vi "ParseXMLRPC.vi"(8 "Parsed In":string, 11 "XML In":string) -> (0 "Parsed Out":string, 3 "XML Out":string)   [LabVIEW 2012]
panel:
  # "<value><array><data>\n  <value>test</value>\n  <value><boolean>1</boolean></value>\n</data></array></value>"
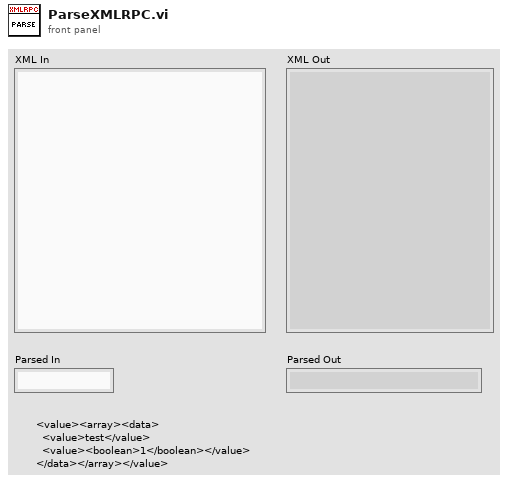
[diagram p1: front panel]
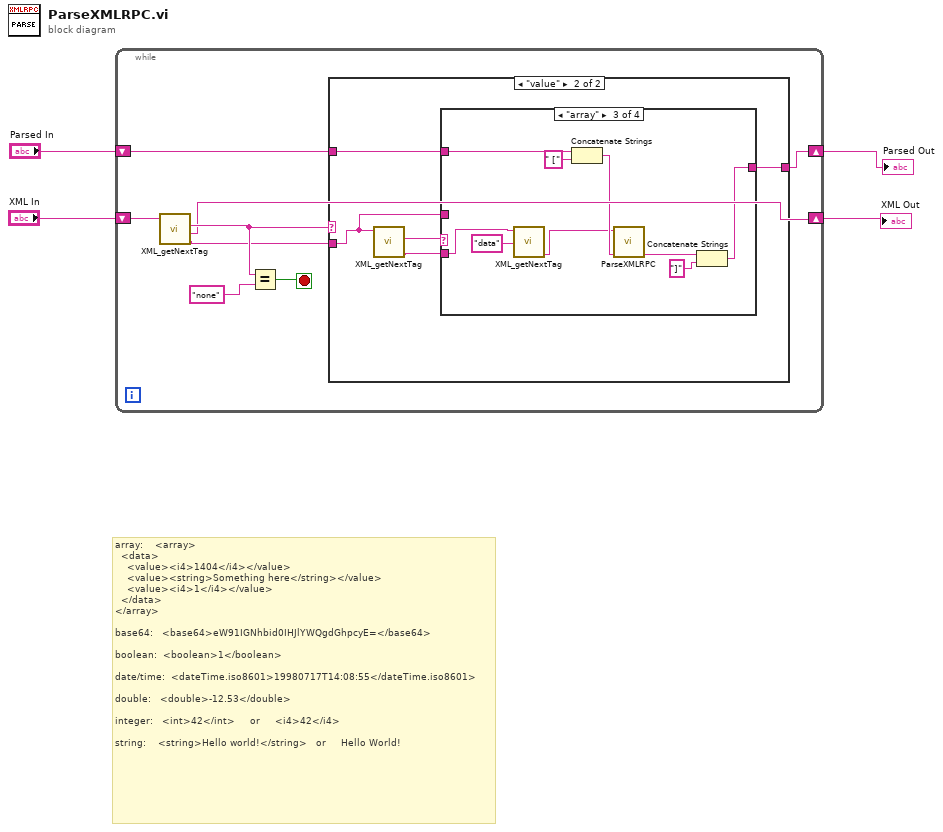
[diagram p0: block diagram]
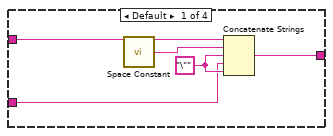
[diagram p3: hidden frame]
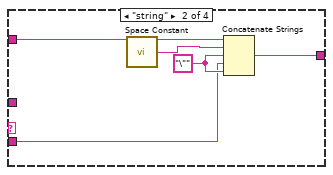
[diagram p4: hidden frame]
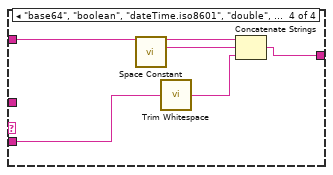
[diagram p5: hidden frame]
diagram:
  # "array:    <array>\n  <data>\n    <value><i4>1404</i4></value>\n    <value><string>Something here</string></value>\n    <value><i4>1</i4></value>\n  </data>\n</array>\n\nbase64:   <base64>eW91IGNhbid0IHJlYWQgdGhpcyE=</base64>\n\nboolean:  <boolean>1</boolean> \n\ndate/time:  <dateTime.iso8601>19980717T14:08:55</dateTime.iso8601>\n\ndouble:   <double>-12.53</double>\n\ninteger:   <int>42</int>     or     <i4>42</i4>\n\nstring:    <string>Hello world!</string>   or     Hello World!"
  n1 = while {
    shift-right: [w7] -> w1
    shift-left: "XML In" -> [w5]
    shift-right: [w11] -> w2
    shift-left: "Parsed In" -> [w12]
    stop <- w10 stop-if-true
    n2 = call <userlib>:"XML_getNextTag.vi"("XML in"=w5) -> ("Value"=w6:string, "after Tag"=w7:string, "Tag Found"=w8:string)  [unwired: 7 in, 1 out]
    n3 = Equal?(x=w8, y="none") -> (x = y?=w10:bool)
    n4 = case shown="\"value\"" w8 {
      tunnel: w6 -> [_ w16]
      tunnel: w12 -> [w13 w18]
      tunnel: [w13 w17] -> w11
      frame Default {
      }
      frame "value" {
        n5 = call <userlib>:"XML_getNextTag.vi"("XML in"=w16) -> ("Value"=w14:string, "Tag Found"=w15:string)  [unwired: 7 in, 2 out]
        n6 = case shown="\"array\"" w15 {
          tunnel: w16 -> [w21 _ _ _]
          tunnel: w14 -> [_ w25 w30 w42]
          tunnel: w18 -> [w23 w28 w37 w40]
          tunnel: [w20 w26 w32 w38] -> w17
          frame Default {
            w22 = "\"" ("string")
            n7 = call <vilib>:"Space Constant.vi"() -> ("String"=w19:string)
            n8 = Concatenate Strings(w23, w19, w22, w21, w22) -> (w20:string)
          }
          frame "string" {
            w27 = "\"" ("string")
            n9 = call <vilib>:"Space Constant.vi"() -> ("String"=w24:string)
            n10 = Concatenate Strings(w28, w24, w27, w25, w27) -> (w26:string)
          }
          frame "array" {
            n11 = call <userlib>:"XML_getNextTag.vi"("Tag"="data", "XML in"=w30) -> ("Value"=w29:string)  [unwired: 6 in, 3 out]
            n12 = Concatenate Strings(w37, " [" ("string")) -> (w35:string)
            n13 = call <userlib>:"ParseXMLRPC.vi"("Parsed In"=w35, "XML In"=w29) -> ("Parsed Out"=w34:string)  [unwired: 8 in, 1 out]
            n14 = Concatenate Strings(w34, "]" ("string")) -> (w32:string)
          }
          frame "base64", "boolean", "dateTime.iso8601", "double", "i4", "int" {
            n15 = call <vilib>:"Space Constant.vi"() -> ("String"=w41:string)
            n16 = call <vilib>:"Trim Whitespace.vi"("string"=w42) -> ("trimmed string"=w39:string)  [unwired: 1 in]
            n17 = Concatenate Strings(w40, w41, w39) -> (w38:string)
          }
        }
      }
    }
  }
  "XML Out" <- w1
  "Parsed Out" <- w2
